vi "Koheras_Configuration.vi"(0 "laserPower":i32=20, 5 "error in":errorcluster) -> (19 "out":errorcluster)   [LabVIEW 2011]
uses:
  Variables/LaserParameter.vi
  Utilities/globalvariables/KoherasGetSetStatus.vi
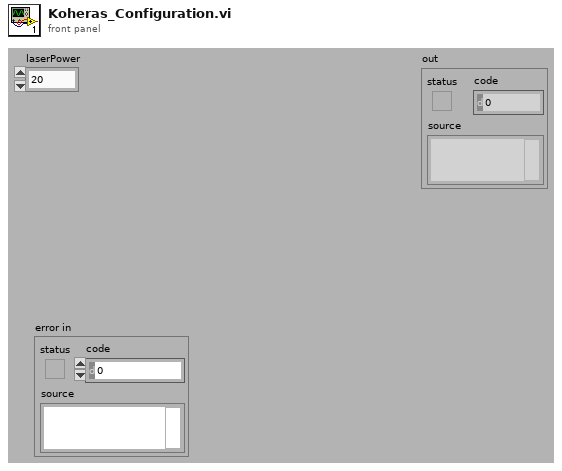
[diagram p1: front panel]
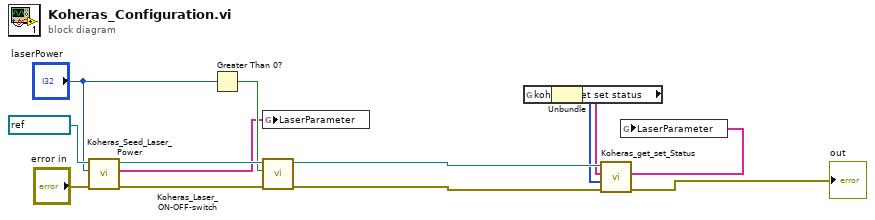
[diagram p0: block diagram]
diagram:
  n1 = call "Koheras_Seed_Laser_Power.vi"("error in"="error in", "laserPower"="laserPower", "VISA resource name in"=refnum<visa-resource-name> "COM3") -> ("error out"=w6:errorcluster, "Return"=w8:string[], "VISA resource name out"=w13:refnum<visa-resource-name>)  [unwired: 6 in]
  n2 = Greater Than 0?(x="laserPower") -> (x > 0?=w10:bool)
  n3 = global write "LaserParameter.vi" "LaserParameter"(w8) -> ()
  n4 = call "Koheras_Laser_ON-OFF-switch.vi"("error in"=w6, "Koheras Seed Laser"=w10, "VISA resource name in"=w13) -> ("error out"=w4:errorcluster, "VISA resource name out"=w14:refnum<visa-resource-name>)  [unwired: 6 in, 1 out]
  n5 = global read "KoherasGetSetStatus.vi" "koheras get set status"() -> (w3:cluster{string[], i32[]})
  n6 = Unbundle(w3) -> (w2:string[], w1:i32[])
  n7 = call "Koheras_get_set_Status.vi"("error in"=w4, "Array 2"=w1, "Array"=w2, "VISA resource name in"=w14) -> ("error out"=→"out":errorcluster, "Return"=w7:string[])  [unwired: 5 in, 1 out]
  n8 = global write "LaserParameter.vi" "LaserParameter"(w7) -> ()
